vi "helper - Plot Polar Data.vi"(4 "Size":u16, 5 "Lines/Points":enum16{"Lines", "Points"}(ring)=enum."Points", 6 "polar attributes":T2 {"minimum" format="%0.2f"; "maximum" format="%0.2f"}, 7 "grid measurements":T1 {"end angle" format="%0.2f"; "start angle" format="%0.2f"; "scale factors"."b" format="%0.2f"; "scale factors"."a" format="%0.2f"}, 8 "polar data":cluster{"magnitude":dbl, "phase":dbl}[](array[cluster]) {"phase" format="%0.2f"; "magnitude" format="%0.2f"}, 9 "picture":picture) -> (3 "new picture":picture)   [LabVIEW 2011]
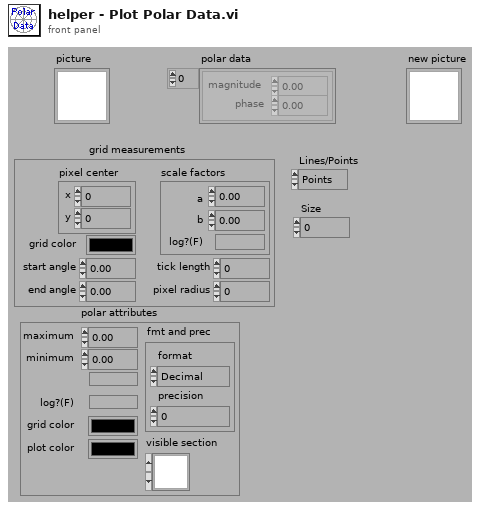
[diagram p1: front panel]
types:
  T1 = cluster{"pixel center":cluster{"x":i16, "y":i16}, "scale factors":cluster{"a":dbl, "b":dbl, "log?(F)":bool}, "grid color":u32, "start angle":dbl, "end angle":dbl, "tick length":i16, "pixel radius":i32}
  T2 = cluster{"maximum":dbl, "minimum":dbl, "clip to min":bool, "log?(F)":bool, "grid color":u32, "plot color":u32, "fmt and prec":cluster{"format":enum8{"Decimal", "Scientific", "Engineering", "Binary", "Octal", "Hex"}, "precision":u8}, "visible section":u16}
  T3 = enum32{"Solid", "Dash", "Dot", "DashDot", "DashDotDot"}
  T4 = cluster{"Size":u16, "Style":enum32{"Solid", "Dash", "Dot", "DashDot", "DashDotDot"}}
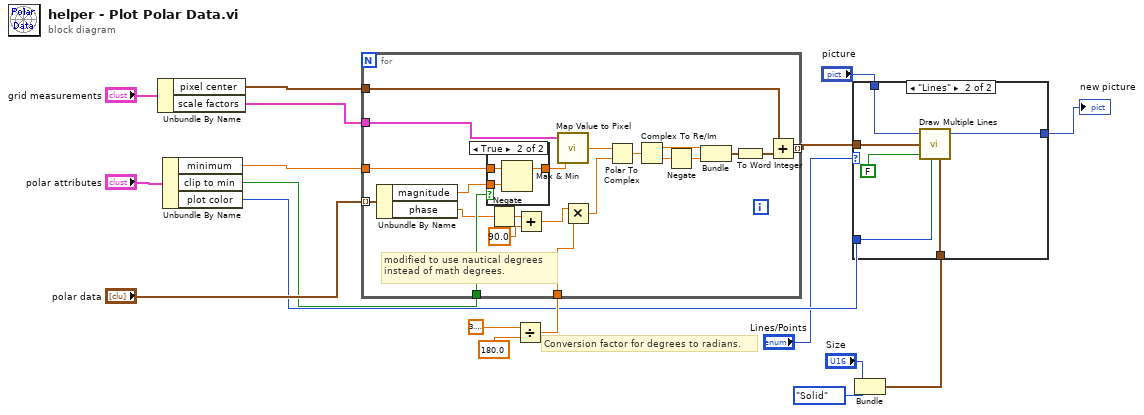
[diagram p0: block diagram]
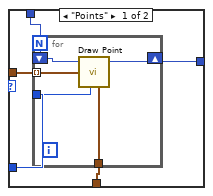
[diagram p2: hidden frame]
diagram:
  # "Conversion factor for degrees to radians."
  n1 = Unbundle By Name("grid measurements") -> ("pixel center"=w14:cluster{"x":i16, "y":i16}, "scale factors"=w15:cluster{"a":dbl, "b":dbl, "log?(F)":bool})
  n2 = Unbundle By Name("polar attributes") -> ("minimum"=w13:dbl, "clip to min"=w12:bool, "plot color"=w7:u32)
  n3 = Divide(x=3.141592653589793, y=180.0) -> (x/y=w10:dbl)
  n4 = for {
    tunnel: "polar data" -> [w39] mode=indexing
    tunnel: w14 -> [w38]
    tunnel: [w37] -> w8 mode=indexing
    tunnel: w15 -> [w30]
    tunnel: w13 -> [w26]
    tunnel: w12 -> [w25]
    tunnel: w10 -> [w23]
    # "modified to use nautical degrees\ninstead of math degrees."
    n5 = Unbundle By Name(w39) -> ("magnitude"=w27:dbl, "phase"=w20:dbl)
    n6 = case shown="True" w25 {
      tunnel: w27 -> [w40 w43]
      tunnel: [w40 w42] -> w28
      tunnel: w26 -> [_ w41]
      frame False {
      }
      frame True {
        n7 = Max & Min(x=w41, y=w43) -> (max(x,y)=w42:dbl)  [unwired: 1 out]
      }
    }
    n8 = Negate(x=w20) -> (-x=w22:dbl)
    n9 = Add(x=w22, y=90.0) -> (x+y=w19:dbl)
    n10 = call <vilib>:"Map Value to Pixel.vi"("x"=w28, "scale factors"=w30) -> ("pixel"=w29:dbl)  [unwired: 1 out]
    n11 = Multiply(x=w19, y=w23) -> (x*y=w24:dbl)
    n12 = Polar To Complex(1:w24, 2:w29) -> (0:w36:cdb)
    n13 = Complex To Re/Im(x + iy=w36) -> (x=w34:dbl, y=w33:dbl)
    n14 = Negate(x=w33) -> (-x=w31:dbl)
    n15 = Bundle(w34, w31) -> (w35:cluster{dbl, dbl})  [unwired: 1 out]
    n16 = To Word Integer(number=w35) -> (16bit integer=w32:cluster{i16, i16})
    n17 = Add(x=w38, y=w32) -> (x+y=w37:cluster{i16, i16})
  }
  n18 = Bundle("Size"="Size", "Style"=T3."Solid") -> (w1:T4)  [unwired: 1 in]
  n19 = case shown="\"Lines\"" "Lines/Points" {
    tunnel: w8 -> [w48 w58]
    tunnel: w7 -> [w45 w57]
    tunnel: [w46 w56] -> w6
    tunnel: "picture" -> [w47 w55]
    tunnel: w1 -> [w44 w54]
    frame "Points" {
      n20 = for {
        tunnel: w48 -> [w53] mode=indexing
        shift-right: [w51] -> w46
        shift-left: w47 -> [w52]
        tunnel: w45 -> [w50]
        tunnel: w44 -> [w49]
        n21 = call <vilib>:"Draw Point.vi"("picture"=w52, "point(x,y)"=w53, "color(black)"=w50, "pen"=w49) -> ("new picture"=w51:picture)  [unwired: 5 out]
      }
    }
    frame "Lines" {
      n22 = call <vilib>:"Draw Multiple Lines.vi"("picture"=w55, "line endpoints"=w58, "fill?(F)"=FALSE, "color(black)"=w57, "pen"=w54) -> ("new picture"=w56:picture)  [unwired: 4 out]
    }
  }
  "new picture" <- w6
